vi "Call.vi"(8 "error in (no error)":errorcluster, 9 "Parameter":variant, 10 "Function":string, 11 "input in":refnum<class "input.lvclass">) -> (0 "error out":errorcluster, 2 "result":refnum<class "result_from_call.lvclass">, 3 "input out":refnum<class "input.lvclass">)   [LabVIEW 2015, in "input.lvclass"]
uses:
  input.lvclass
  Result/result_from_call/result_from_call.lvclass
  input.lvclass/input.ctl
  <vilib>/addons/lv-msgpack/MsgPack Serializer/MsgPackSerializer.lvclass
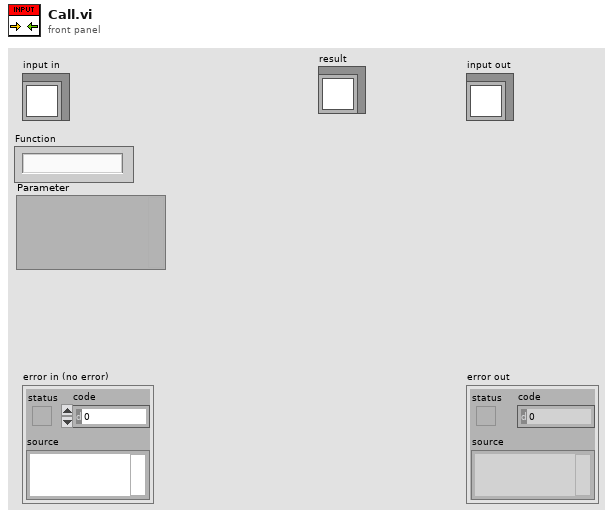
[diagram p1: front panel]
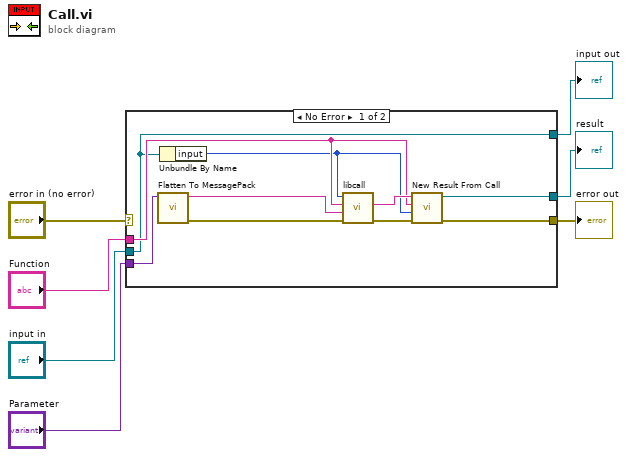
[diagram p0: block diagram]
diagram:
  n1 = case shown="No Error" "error in (no error)" {
    selector: "error in (no error)" -> [_ w19]
    tunnel: [w11 w19] -> w6
    tunnel: [w9 w18] -> w4
    tunnel: "input in" -> [w9 w18]
    tunnel: "Parameter" -> [w17 _]
    tunnel: "Function" -> [w13 _]
    tunnel: [w10 _] -> w1
    frame No Error {
      n2 = call <vilib>:"Flatten To MessagePack.vi"("Data"=w17) -> ("error out"=w16:errorcluster, "MsgPack Data"=w15:string)  [unwired: 9 in]
      n3 = Unbundle By Name(w9) -> ("input"=w8:i32)
      n4 = call "libcall.vi"("error in (no error)"=w16, "Parameter"=w15, "Function"=w13, "input"=w8) -> ("error out"=w12:errorcluster, "id"=w14:string)  [unwired: 6 in]
      n5 = call "New Result From Call.vi"("error in (no error)"=w12, "input"=w8, "function"=w13, "id"=w14) -> ("error out"=w11:errorcluster, "result"=w10:refnum<class "result_from_call.lvclass">)  [unwired: 6 in]
    }
    frame Error {
    }
  }
  "error out" <- w6
  "input out" <- w4
  "result" <- w1
